vi "GetAllVIs.vi"(11 "onlyOpen":bool) -> (0 "errorOut":string, 3 "VIs in memory":T1[](array[typedef]))   [LabVIEW 2009]
uses:
  <vilib>/Utility/allVIsInMemory.llb/VIMemory VI info.ctl
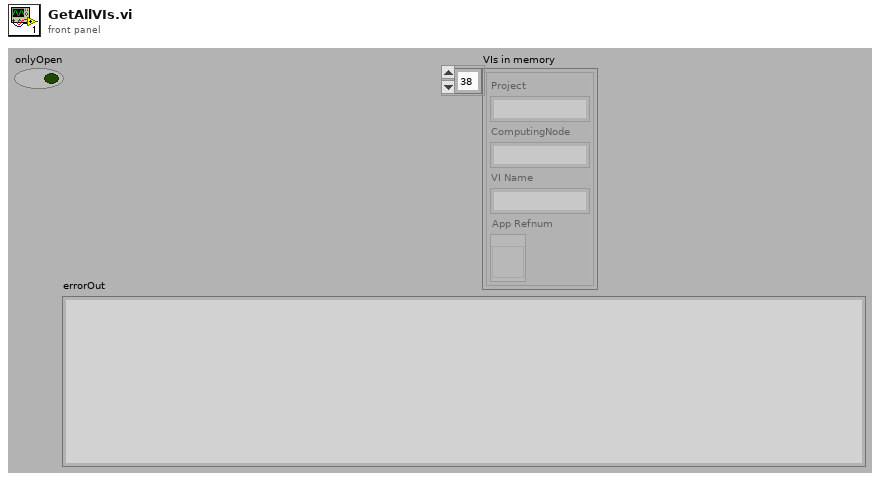
[diagram p1: front panel]
types:
  T1 = typedef "VIMemory VI info.ctl" = cluster{"Project":string, "ComputingNode":string, "VI Name":string, "App Refnum":refnum<vi>}
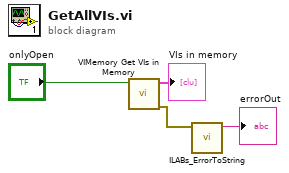
[diagram p0: block diagram]
diagram:
  n1 = call <vilib>:"VIMemory Get VIs in Memory.vi"("Only VIs with Open FPs?"="onlyOpen") -> ("error out"=w2:errorcluster, "VIs in memory"=→"VIs in memory":T1[])  [unwired: 1 in, 8 out]
  n2 = call "ILABs_ErrorToString.vi"("errorIn"=w2) -> ("errorOut"=→"errorOut":string)  [unwired: 10 out]
